vi "StiffbackGluing.vi"() -> ()   [LabVIEW 2015]
uses:
  GlobalPath.vi
  GlobalData.vi
  GlobalVi.vi
panel:
  in  "ptfe 12":bool caption="Manually distribute glue on external area"
  in  "ptfe 9":bool caption="Position the cartridge on the glue machine housing"
  out "PanelName":string
  in  "DONE ALL?":bool
  in  "ptfe 10":bool caption="Remove parchment protections"
  in  "ptfe 8":bool caption="Mount the dispenser on the glue cartridge"
  in  "ptfe 7":bool caption="Position parchment covers to protect the stiffback plates and external\nparts of the 5 PCBs"
  in  "Done with gluing?":bool
  in  "ptfe 5":bool caption="Open the vi with the gluing instructions"
  in  "ptfe 4":bool caption="Release stiffback from the movement arch and move arch away"
  in  "ptfe 2":bool caption="Position stiffback face up on table"
  # "1. Gluing on Stiffback"
  # "2. Start gluing process"
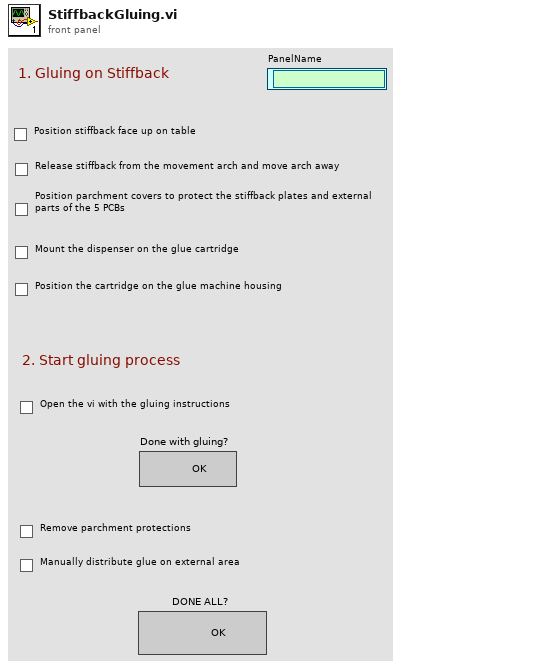
[diagram p1: front panel]
types:
  T1 = enum16{"open", "replace", "create", "open or create", "replace or create", "replace or create with confirmation"}
  T2 = enum32{"Bad", "Idle", "Run top level", "Running"}
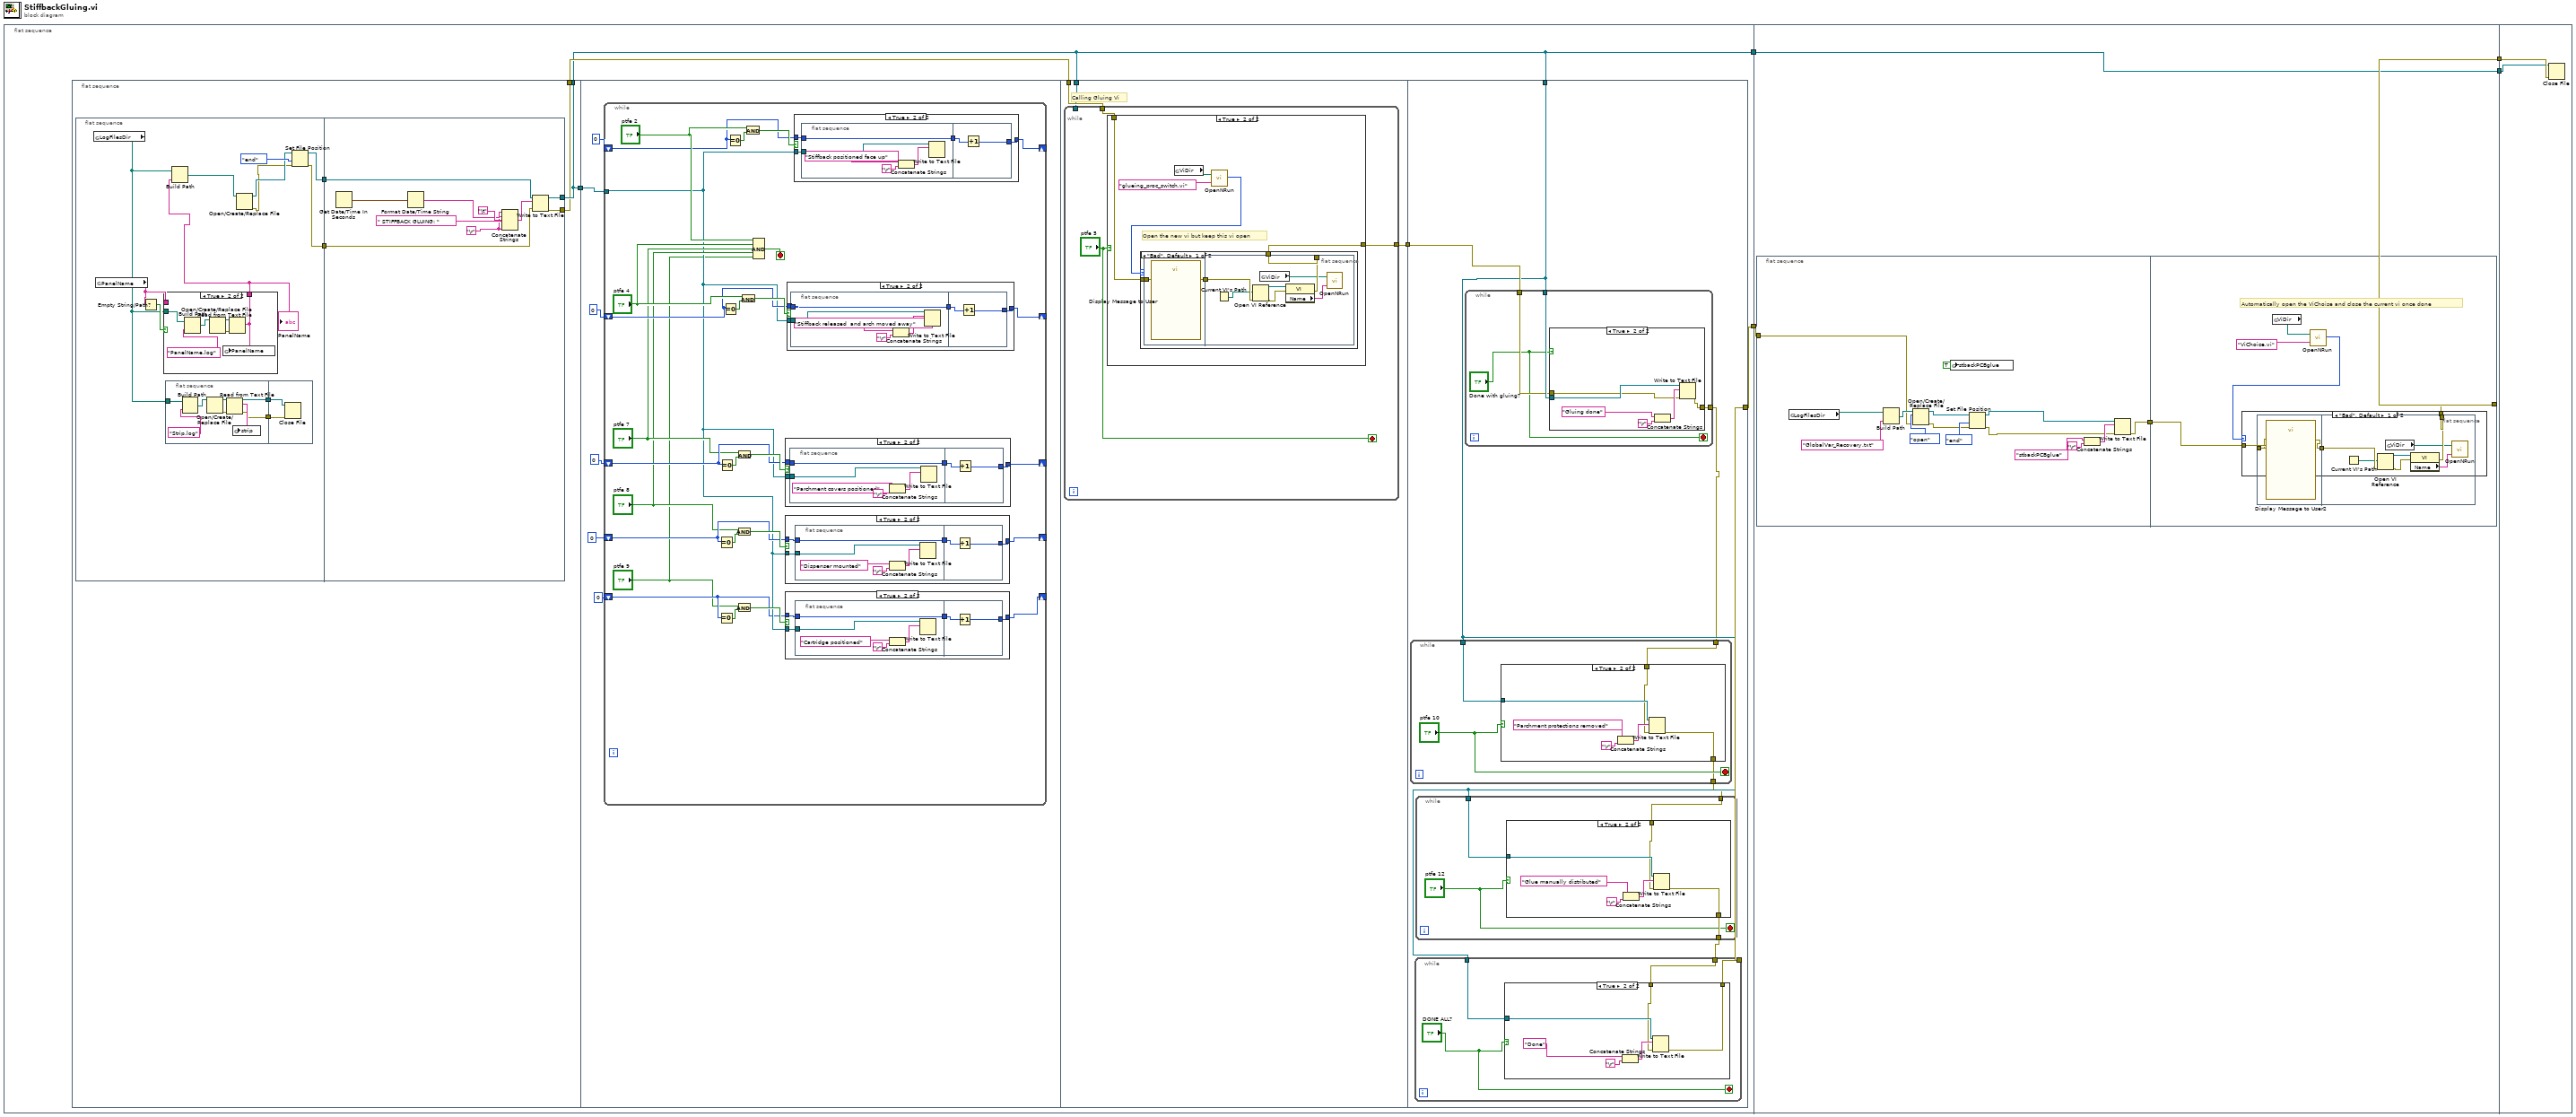
[diagram p0: block diagram]
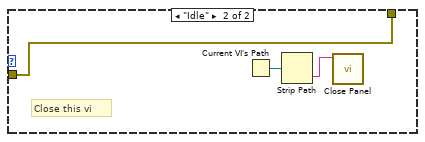
[diagram p14: hidden frame]
diagram:
  n1 = flat-sequence {
    tunnel: [w6] -> w3
    tunnel: [w5] -> w1
    tunnel: [w224] -> w4
    tunnel: w3 -> [w223]
    tunnel: [w223] -> w2
    tunnel: w1 -> [w221]
    tunnel: w4 -> [w261]
    tunnel: w2 -> [w260]
    frame #0 {
      n2 = flat-sequence {
        tunnel: [w12] -> w9
        tunnel: [w12] -> w6
        tunnel: [w11] -> w8
        tunnel: w9 -> [w58]
        tunnel: w8 -> [w148]
        tunnel: w6 -> [w146]
        tunnel: [w147] -> w7
        tunnel: w7 -> [w176]
        tunnel: w6 -> [w174]
        tunnel: [w175] -> w5
        frame #0 {
          n3 = flat-sequence {
            tunnel: [w20] -> w13
            tunnel: [w21] -> w10
            tunnel: w13 -> [w48]
            tunnel: [w47] -> w12
            tunnel: [w46] -> w11
            tunnel: w10 -> [w45]
            frame #0 {
              n4 = global read "GlobalPath.vi" "LogFilesDir"() -> (w14:path)
              n5 = global read "GlobalData.vi" "PanelName"() -> (w19:string)
              n6 = Empty String/Path?(string/path=w19) -> (empty?=w18:bool)
              n7 = case shown="True" w18 {
                tunnel: w14 -> [_ w42]
                tunnel: [w36 w37] -> w17
                tunnel: w19 -> [w36 _]
                frame False {
                }
                frame True {
                  n8 = Build Path(base path=w42, name or relative path="PanelName.log") -> (appended path=w41:path)
                  n9 = Open/Create/Replace File(file path (use dialog)=w41) -> (refnum out=w38:refnum<file>, error out=w39:errorcluster)  [unwired: 5 in, 1 out]
                  n10 = Read from Text File(file (use dialog)=w38, error in=w39) -> (text=w37:string)  [unwired: 2 in, 3 out]
                  n11 = global write "GlobalData.vi" "PanelName"(w37) -> ()
                }
              }
              "PanelName" <- w17
              n12 = flat-sequence {
                tunnel: w14 -> [w33]
                tunnel: [w27] -> w16
                tunnel: [w26] -> w15
                tunnel: w16 -> [w35]
                tunnel: w15 -> [w34]
                frame #0 {
                  n13 = Build Path(base path=w33, name or relative path="Strip.log") -> (appended path=w32:path)
                  n14 = Open/Create/Replace File(file path (use dialog)=w32) -> (refnum out=w29:refnum<file>, error out=w30:errorcluster)  [unwired: 5 in, 1 out]
                  n15 = Read from Text File(file (use dialog)=w29, error in=w30) -> (refnum out=w26:refnum<file>, text=w28:string, error out=w27:errorcluster)  [unwired: 2 in, 1 out]
                  n16 = global write "GlobalData.vi" "strip"(w28) -> ()
                }
                frame #1 {
                  n17 = Close File(refnum=w34, error in=w35) -> ()  [unwired: 2 out]
                }
              }
              n18 = Build Path(base path=w14, name or relative path=w17) -> (appended path=w25:path)
              n19 = Open/Create/Replace File(file path (use dialog)=w25) -> (refnum out=w23:refnum<file>, error out=w22:errorcluster)  [unwired: 5 in, 1 out]
              n20 = Set File Position(refnum=w23, from (0:start)=enum16{"start", "end", "current"}."end", error in=w22) -> (refnum out=w20:refnum<file>, error out=w21:errorcluster)  [unwired: 1 in]
            }
            frame #1 {
              w43 = "\r"
              n21 = Get Date/Time In Seconds() -> (seconds since 1Jan1904=w44:timestamp)
              n22 = Format Date/Time String(seconds (now)=w44) -> (date/time string=w50:string)  [unwired: 2 in]
              n23 = Concatenate Strings(w43, w50, "\t", " STIFFBACK GLUING: ", w43) -> (w49:string)
              n24 = Write to Text File(file (use dialog)=w48, text=w49, error in=w45) -> (refnum out=w47:refnum<file>, error out=w46:errorcluster)  [unwired: 1 in, 1 out]
            }
          }
        }
        frame #1 {
          n25 = while {
            tunnel: w58 -> [w62]
            shift-right: [w80] -> _
            shift-left: 0 -> [w81]
            shift-right: [w75] -> _
            shift-left: 0 -> [w76]
            shift-right: [w71] -> _
            shift-left: 0 -> [w72]
            shift-right: [w65] -> _
            shift-left: 0 -> [w67]
            shift-right: [w60] -> _
            shift-left: 0 -> [w61]
            stop <- w85 stop-if-true
            n26 = Equal To 0?(x=w67) -> (x = 0?=w69:bool)
            n27 = Equal To 0?(x=w61) -> (x = 0?=w64:bool)
            n28 = Equal To 0?(x=w72) -> (x = 0?=w74:bool)
            n29 = Equal To 0?(x=w76) -> (x = 0?=w79:bool)
            n30 = Equal To 0?(x=w81) -> (x = 0?=w84:bool)
            n31 = And(x="ptfe 8", y=w69) -> (x .and. y?=w68:bool)
            n32 = And(x="ptfe 9", y=w64) -> (x .and. y?=w63:bool)
            n33 = And(x="ptfe 7", y=w74) -> (x .and. y?=w73:bool)
            n34 = And(x="ptfe 4", y=w79) -> (x .and. y?=w78:bool)
            n35 = And(x="ptfe 2", y=w84) -> (x .and. y?=w83:bool)
            n36 = Compound Arithmetic op=AND("ptfe 2", "ptfe 4", "ptfe 7", "ptfe 8", "ptfe 9") -> (w85:bool)
            n37 = case shown="True" w68 {
              tunnel: w62 -> [_ w102]
              tunnel: w67 -> [w98 w100]
              tunnel: [w98 w99] -> w65
              frame False {
              }
              frame True {
                n38 = flat-sequence {
                  tunnel: w102 -> [w105]
                  tunnel: [w104] -> w101
                  tunnel: w100 -> [w104]
                  tunnel: w101 -> [w109]
                  tunnel: [w108] -> w99
                  frame #0 {
                    n39 = Concatenate Strings("Dispenser mounted", "\r") -> (w107:string)
                    n40 = Write to Text File(file (use dialog)=w105, text=w107) -> ()  [unwired: 2 in, 3 out]
                  }
                  frame #1 {
                    n41 = Increment(x=w109) -> (x+1=w108:i32)
                  }
                }
              }
            }
            n42 = case shown="True" w63 {
              tunnel: w62 -> [_ w90]
              tunnel: w61 -> [w86 w88]
              tunnel: [w86 w87] -> w60
              frame False {
              }
              frame True {
                n43 = flat-sequence {
                  tunnel: w90 -> [w93]
                  tunnel: [w92] -> w89
                  tunnel: w88 -> [w92]
                  tunnel: w89 -> [w97]
                  tunnel: [w96] -> w87
                  frame #0 {
                    n44 = Concatenate Strings("Cartridge positioned", "\r") -> (w95:string)
                    n45 = Write to Text File(file (use dialog)=w93, text=w95) -> ()  [unwired: 2 in, 3 out]
                  }
                  frame #1 {
                    n46 = Increment(x=w97) -> (x+1=w96:i32)
                  }
                }
              }
            }
            n47 = case shown="True" w73 {
              tunnel: w62 -> [_ w114]
              tunnel: w72 -> [w110 w112]
              tunnel: [w110 w111] -> w71
              frame False {
              }
              frame True {
                n48 = flat-sequence {
                  tunnel: w114 -> [w117]
                  tunnel: [w116] -> w113
                  tunnel: w112 -> [w116]
                  tunnel: w113 -> [w121]
                  tunnel: [w120] -> w111
                  frame #0 {
                    n49 = Concatenate Strings("Parchment covers positioned", "\r") -> (w119:string)
                    n50 = Write to Text File(file (use dialog)=w117, text=w119) -> ()  [unwired: 2 in, 3 out]
                  }
                  frame #1 {
                    n51 = Increment(x=w121) -> (x+1=w120:i32)
                  }
                }
              }
            }
            n52 = case shown="True" w78 {
              tunnel: w62 -> [_ w126]
              tunnel: w76 -> [w122 w124]
              tunnel: [w122 w123] -> w75
              frame False {
              }
              frame True {
                n53 = flat-sequence {
                  tunnel: w126 -> [w129]
                  tunnel: [w128] -> w125
                  tunnel: w124 -> [w128]
                  tunnel: w125 -> [w133]
                  tunnel: [w132] -> w123
                  frame #0 {
                    n54 = Concatenate Strings("Stiffback released  and arch moved away", "\r") -> (w131:string)
                    n55 = Write to Text File(file (use dialog)=w129, text=w131) -> ()  [unwired: 2 in, 3 out]
                  }
                  frame #1 {
                    n56 = Increment(x=w133) -> (x+1=w132:i32)
                  }
                }
              }
            }
            n57 = case shown="True" w83 {
              tunnel: w62 -> [_ w138]
              tunnel: w81 -> [w134 w136]
              tunnel: [w134 w135] -> w80
              frame False {
              }
              frame True {
                n58 = flat-sequence {
                  tunnel: w138 -> [w141]
                  tunnel: [w140] -> w137
                  tunnel: w136 -> [w140]
                  tunnel: w137 -> [w145]
                  tunnel: [w144] -> w135
                  frame #0 {
                    n59 = Concatenate Strings("Stiffback positioned face up", "\r") -> (w143:string)
                    n60 = Write to Text File(file (use dialog)=w141, text=w143) -> ()  [unwired: 2 in, 3 out]
                  }
                  frame #1 {
                    n61 = Increment(x=w145) -> (x+1=w144:i32)
                  }
                }
              }
            }
          }
        }
        frame #2 {
          # "Calling Gluing Vi"
          n62 = while {
            tunnel: w148 -> [w151]
            tunnel: [w150] -> w147
            tunnel: w146 -> [_]
            stop <- "ptfe 5" stop-if-true
            n63 = case shown="True" "ptfe 5" {
              tunnel: w151 -> [w152 w154]
              tunnel: [w152 w153] -> w150
              frame False {
              }
              frame True {
                # "Open the new vi but keep this vi open"
                n64 = global read "GlobalPath.vi" "ViDir"() -> (w157:path)
                n65 = call "OpenNRun.vi"("VI name"="glueing_proc_switch.vi", "ViDirPath"=w157) -> ("Execution:State"=w156:T2)
                n66 = case shown="\"Bad\", Default" w156 {
                  tunnel: [w160 w170] -> w153
                  tunnel: w154 -> [w159 w170]
                  frame "Bad", Default {
                    n67 = flat-sequence {
                      tunnel: w159 -> [w161]
                      tunnel: [w162] -> w158
                      tunnel: [w166] -> w160
                      tunnel: w158 -> [w165]
                      frame #0 {
                        n68 = call "Display Message to User"("error in (no error)"=w161) -> ("error out"=w162:errorcluster)  [unwired: 9 in, 1 out]
                      }
                      frame #1 {
                        n69 = Current VI's Path() -> (path=w163:path)
                        n70 = Open VI Reference(vi path=w163, error in (no error)=w165) -> (vi reference=w169:refnum<vi>, error out=w168:errorcluster)  [unwired: 4 in]
                        n71 = global read "GlobalPath.vi" "ViDir"() -> (w164:path)
                        n72 = property class="VI"(reference=w169, error in=w168) -> (error out=w166:errorcluster, "Name"=w167:string)  [unwired: 1 out]
                        n73 = call "OpenNRun.vi"("VI name"=w167, "ViDirPath"=w164) -> ()  [unwired: 1 out]
                      }
                    }
                  }
                  frame "Idle" {
                    # "Program opened"
                  }
                }
              }
            }
          }
        }
        frame #3 {
          n74 = while {
            tunnel: w174 -> [w213]
            tunnel: [w212] -> w171
            tunnel: w176 -> [w211]
            stop <- "Done with gluing?" stop-if-true
            n75 = case shown="True" "Done with gluing?" {
              tunnel: w213 -> [_ w217]
              tunnel: w211 -> [w214 w216]
              tunnel: [w214 w215] -> w212
              frame False {
              }
              frame True {
                n76 = Concatenate Strings("Gluing done", "\r") -> (w220:string)
                n77 = Write to Text File(file (use dialog)=w217, text=w220, error in=w216) -> (error out=w215:errorcluster)  [unwired: 1 in, 2 out]
              }
            }
          }
          n78 = while {
            tunnel: w171 -> [w202]
            tunnel: w174 -> [w201]
            tunnel: [w199] -> w173
            stop <- "ptfe 10" stop-if-true
            n79 = case shown="True" "ptfe 10" {
              tunnel: w202 -> [w203 w205]
              tunnel: w201 -> [_ w206]
              tunnel: [w203 w204] -> w199
              frame False {
              }
              frame True {
                n80 = Concatenate Strings("Parchment protections removed", "\r") -> (w209:string)
                n81 = Write to Text File(file (use dialog)=w206, text=w209, error in=w205) -> (error out=w204:errorcluster)  [unwired: 1 in, 2 out]
              }
            }
          }
          n82 = while {
            tunnel: w173 -> [w180]
            tunnel: w174 -> [w179]
            tunnel: [w178] -> w172
            stop <- "ptfe 12" stop-if-true
            n83 = case shown="True" "ptfe 12" {
              tunnel: w180 -> [w181 w183]
              tunnel: w179 -> [_ w184]
              tunnel: [w181 w182] -> w178
              frame False {
              }
              frame True {
                n84 = Concatenate Strings("Glue manually distributed", "\r") -> (w187:string)
                n85 = Write to Text File(file (use dialog)=w184, text=w187, error in=w183) -> (error out=w182:errorcluster)  [unwired: 1 in, 2 out]
              }
            }
          }
          n86 = while {
            tunnel: w172 -> [w191]
            tunnel: w174 -> [w190]
            tunnel: [w189] -> w175
            stop <- "DONE ALL?" stop-if-true
            n87 = case shown="True" "DONE ALL?" {
              tunnel: w191 -> [w192 w194]
              tunnel: w190 -> [_ w195]
              tunnel: [w192 w193] -> w189
              frame False {
              }
              frame True {
                n88 = Concatenate Strings("Done", "\r") -> (w198:string)
                n89 = Write to Text File(file (use dialog)=w195, text=w198, error in=w194) -> (error out=w193:errorcluster)  [unwired: 1 in, 2 out]
              }
            }
          }
        }
      }
    }
    frame #1 {
      n90 = flat-sequence {
        tunnel: [w228] -> w222
        tunnel: w221 -> [w227]
        tunnel: [w241] -> w224
        tunnel: w222 -> [w240]
        frame #0 {
          n91 = global read "GlobalPath.vi" "LogFilesDir"() -> (w225:path)
          n92 = Build Path(base path=w225, name or relative path="GlobalVar_Recovery.txt") -> (appended path=w237:path)
          n93 = Open/Create/Replace File(file path (use dialog)=w237, error in=w227, operation (0:open)=T1."open") -> (refnum out=w233:refnum<file>, error out=w234:errorcluster)  [unwired: 3 in, 1 out]
          n94 = global write "GlobalVi.vi" "stbackPCBglue"(TRUE) -> ()
          n95 = Set File Position(refnum=w233, from (0:start)=enum16{"start", "end", "current"}."end", error in=w234) -> (refnum out=w230:refnum<file>, error out=w229:errorcluster)  [unwired: 1 in]
          n96 = Concatenate Strings("stbackPCBglue", "\r") -> (w232:string)
          n97 = Write to Text File(file (use dialog)=w230, text=w232, error in=w229) -> (error out=w228:errorcluster)  [unwired: 1 in, 2 out]
        }
        frame #1 {
          # "Automatically open the ViChoise and close the current vi once done"
          n98 = global read "GlobalPath.vi" "ViDir"() -> (w244:path)
          n99 = call "OpenNRun.vi"("VI name"="ViChoice.vi", "ViDirPath"=w244) -> ("Execution:State"=w243:T2)
          n100 = case shown="\"Bad\", Default" w243 {
            tunnel: [w247 w259] -> w241
            tunnel: w240 -> [w246 w259]
            frame "Bad", Default {
              n101 = flat-sequence {
                tunnel: w246 -> [w249]
                tunnel: [w248] -> w245
                tunnel: [w253] -> w247
                tunnel: w245 -> [w252]
                frame #0 {
                  n102 = call "Display Message to User2"("error in (no error)"=w249) -> ("error out"=w248:errorcluster)  [unwired: 9 in, 1 out]
                }
                frame #1 {
                  n103 = Current VI's Path() -> (path=w250:path)
                  n104 = Open VI Reference(vi path=w250, error in (no error)=w252) -> (vi reference=w256:refnum<vi>, error out=w255:errorcluster)  [unwired: 4 in]
                  n105 = global read "GlobalPath.vi" "ViDir"() -> (w251:path)
                  n106 = property class="VI"(reference=w256, error in=w255) -> (error out=w253:errorcluster, "Name"=w254:string)  [unwired: 1 out]
                  n107 = call "OpenNRun.vi"("VI name"=w254, "ViDirPath"=w251) -> ()  [unwired: 1 out]
                }
              }
            }
            frame "Idle" {
              # "Close this vi"
              n108 = Current VI's Path() -> (path=w258:path)
              n109 = Strip Path(path=w258) -> (name=w257:string)  [unwired: 1 out]
              n110 = call <vilib>:"Close Panel.vi"("VI name"=w257) -> ()  [unwired: 10 in, 1 out]
            }
          }
        }
      }
    }
    frame #2 {
      n111 = Close File(refnum=w260, error in=w261) -> ()  [unwired: 2 out]
    }
  }
